vi "Washing Machine.vi"() -> ()   [LabVIEW 2019]
panel:
  out "Remaining Time (s)":i32 caption="Elapsed Time (s)"
  out "Stage":string
  in  "Mode":u16(ring) items=["Colorful", "Intensive", "Quick Wash", "Select Mode"]
  in  "START":bool
  in  "Turn ON/OFF":bool
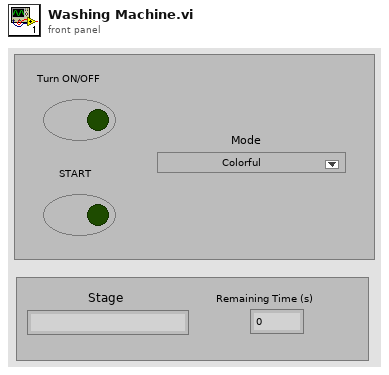
[diagram p1: front panel]
types:
  T1 = enum8{"Enabled", "Disabled", "Disabled and Grayed Out"}
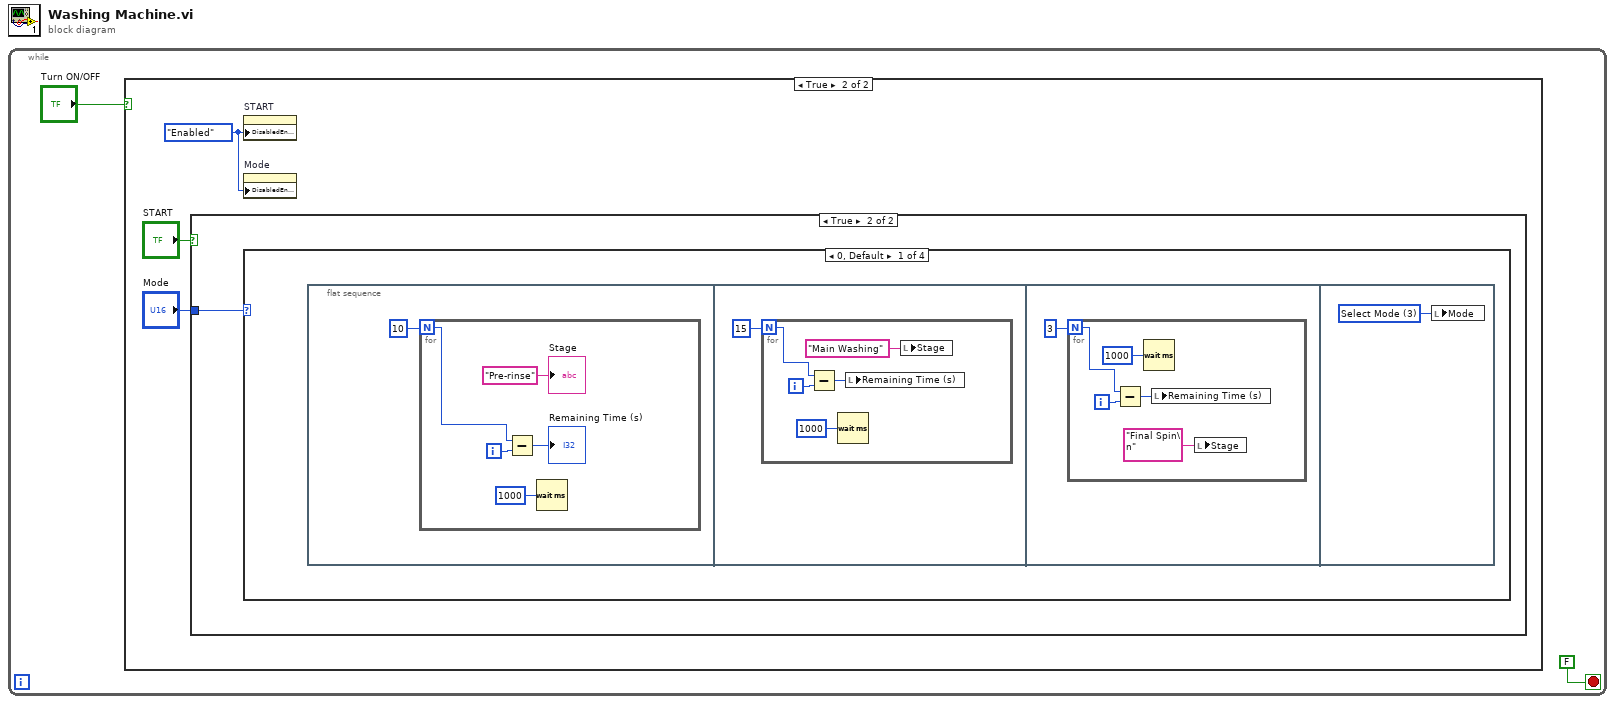
[diagram p0: block diagram]
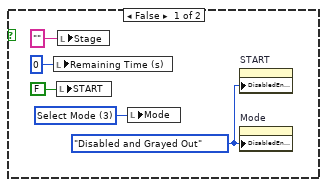
[diagram p2: hidden frame]
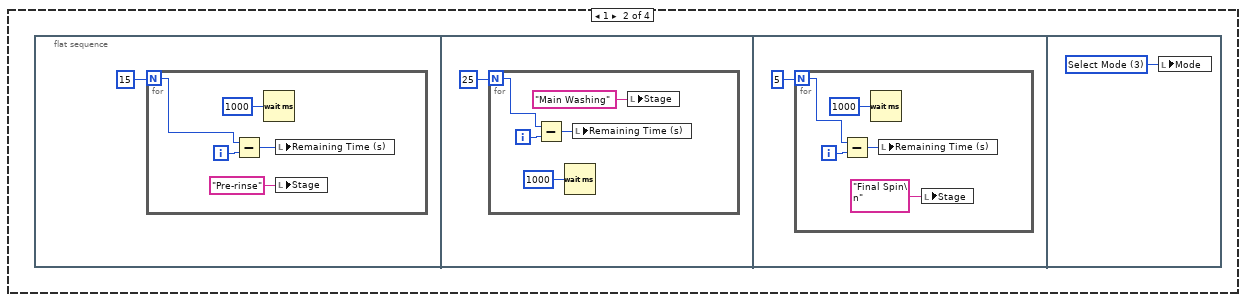
[diagram p4: hidden frame]
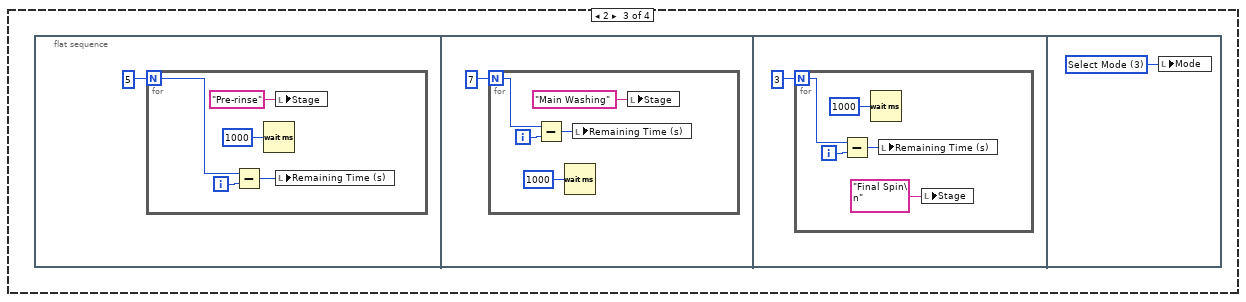
[diagram p5: hidden frame]
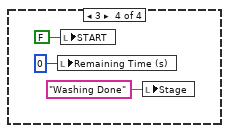
[diagram p6: hidden frame]
diagram:
  n1 = while {
    stop <- FALSE stop-if-true
    n2 = case shown="True" "Turn ON/OFF" {
      frame False {
        w3 = u16 3 items=["Colorful", "Intensive", "Quick Wash", "Select Mode"] ("Mode")
        w7 = T1."Disabled and Grayed Out" ("Disabled")
        n3 = local write "Remaining Time (s)"(0 ("Remaining Time (s)")) -> ()
        n4 = local write "START"(FALSE ("START")) -> ()
        n5 = local write "Stage"("" ("Stage")) -> ()
        n6 = local write "Mode"(w3) -> ()
        n7 = property on="START" class="Bool (strict)"("DisabledEnum"=w7) -> ()  [unwired: 2 in, 2 out]
        n8 = property on="Mode" class="Ring (strict)"("DisabledEnum"=w7) -> ()  [unwired: 2 in, 2 out]
      }
      frame True {
        w8 = T1."Enabled" ("Disabled")
        n9 = case shown="True" "START" {
          tunnel: "Mode" -> [_ w11]
          frame False {
          }
          frame True {
            n10 = case shown="0, Default" w11 {
              frame 0, Default {
                n11 = flat-sequence {
                  frame #0 {
                    n12 = for {
                      N: 10 -> [w14]
                      i -> [w13]
                      n13 = Subtract(x=w14, y=w13) -> (x-y=→"Remaining Time (s)":i32)
                      n14 = Wait (ms)(milliseconds to wait=1000 ("y")) -> ()  [unwired: 1 out]
                      "Stage" <- "Pre-rinse" ("Stage")
                    }
                  }
                  frame #1 {
                    n15 = for {
                      N: 15 -> [w20]
                      i -> [w19]
                      n16 = Subtract(x=w20, y=w19) -> (x-y=w21:i32)
                      n17 = Wait (ms)(milliseconds to wait=1000 ("y")) -> ()  [unwired: 1 out]
                      n18 = local write "Remaining Time (s)"(w21) -> ()
                      n19 = local write "Stage"("Main Washing" ("Stage")) -> ()
                    }
                  }
                  frame #2 {
                    n20 = for {
                      N: 3 -> [w26]
                      i -> [w25]
                      n21 = Subtract(x=w26, y=w25) -> (x-y=w27:i32)
                      n22 = Wait (ms)(milliseconds to wait=1000 ("y")) -> ()  [unwired: 1 out]
                      n23 = local write "Remaining Time (s)"(w27) -> ()
                      n24 = local write "Stage"("Final Spin\n" ("Stage")) -> ()
                    }
                  }
                  frame #3 {
                    w30 = u16 3 items=["Colorful", "Intensive", "Quick Wash", "Select Mode"] ("Mode")
                    n25 = local write "Mode"(w30) -> ()
                  }
                }
              }
              frame 1 {
                n26 = flat-sequence {
                  frame #0 {
                    n27 = for {
                      N: 15 -> [w35]
                      i -> [w34]
                      n28 = Subtract(x=w35, y=w34) -> (x-y=w32:i32)
                      n29 = Wait (ms)(milliseconds to wait=1000 ("y")) -> ()  [unwired: 1 out]
                      n30 = local write "Remaining Time (s)"(w32) -> ()
                      n31 = local write "Stage"("Pre-rinse" ("Stage")) -> ()
                    }
                  }
                  frame #1 {
                    n32 = for {
                      N: 25 -> [w39]
                      i -> [w38]
                      n33 = Subtract(x=w39, y=w38) -> (x-y=w40:i32)
                      n34 = Wait (ms)(milliseconds to wait=1000 ("y")) -> ()  [unwired: 1 out]
                      n35 = local write "Remaining Time (s)"(w40) -> ()
                      n36 = local write "Stage"("Main Washing" ("Stage")) -> ()
                    }
                  }
                  frame #2 {
                    n37 = for {
                      N: 5 -> [w45]
                      i -> [w44]
                      n38 = Subtract(x=w45, y=w44) -> (x-y=w46:i32)
                      n39 = Wait (ms)(milliseconds to wait=1000 ("y")) -> ()  [unwired: 1 out]
                      n40 = local write "Remaining Time (s)"(w46) -> ()
                      n41 = local write "Stage"("Final Spin\n" ("Stage")) -> ()
                    }
                  }
                  frame #3 {
                    w49 = u16 3 items=["Colorful", "Intensive", "Quick Wash", "Select Mode"] ("Mode")
                    n42 = local write "Mode"(w49) -> ()
                  }
                }
              }
              frame 2 {
                n43 = flat-sequence {
                  frame #0 {
                    n44 = for {
                      N: 5 -> [w54]
                      i -> [w53]
                      n45 = Subtract(x=w54, y=w53) -> (x-y=w51:i32)
                      n46 = Wait (ms)(milliseconds to wait=1000 ("y")) -> ()  [unwired: 1 out]
                      n47 = local write "Stage"("Pre-rinse" ("Stage")) -> ()
                      n48 = local write "Remaining Time (s)"(w51) -> ()
                    }
                  }
                  frame #1 {
                    n49 = for {
                      N: 7 -> [w58]
                      i -> [w57]
                      n50 = Subtract(x=w58, y=w57) -> (x-y=w59:i32)
                      n51 = Wait (ms)(milliseconds to wait=1000 ("y")) -> ()  [unwired: 1 out]
                      n52 = local write "Remaining Time (s)"(w59) -> ()
                      n53 = local write "Stage"("Main Washing" ("Stage")) -> ()
                    }
                  }
                  frame #2 {
                    n54 = for {
                      N: 3 -> [w64]
                      i -> [w63]
                      n55 = Subtract(x=w64, y=w63) -> (x-y=w65:i32)
                      n56 = Wait (ms)(milliseconds to wait=1000 ("y")) -> ()  [unwired: 1 out]
                      n57 = local write "Remaining Time (s)"(w65) -> ()
                      n58 = local write "Stage"("Final Spin\n" ("Stage")) -> ()
                    }
                  }
                  frame #3 {
                    w68 = u16 3 items=["Colorful", "Intensive", "Quick Wash", "Select Mode"] ("Mode")
                    n59 = local write "Mode"(w68) -> ()
                  }
                }
              }
              frame 3 {
                n60 = local write "Remaining Time (s)"(0 ("Remaining Time (s)")) -> ()
                n61 = local write "START"(FALSE ("START")) -> ()
                n62 = local write "Stage"("Washing Done" ("Stage")) -> ()
              }
            }
          }
        }
        n63 = property on="START" class="Bool (strict)"("DisabledEnum"=w8) -> ()  [unwired: 2 in, 2 out]
        n64 = property on="Mode" class="Ring (strict)"("DisabledEnum"=w8) -> ()  [unwired: 2 in, 2 out]
      }
    }
  }
